vi "13_EventLogger_callback.vi"(4 "String":refnum<vi>, 5 "Event Data":cluster{"level":i32, "message":string}, 6 "Control Ref":refnum<k24>, 7 "Event Common Data":T1) -> ()   [LabVIEW 2014]
uses:
  SwabianInstruments.TimeTagger
panel:
  # "This is a callback VI that LabView will call automatically on each \ncaptured .NET Event.\n\nYou can create this VI by right clicking on \"VI Ref\" field of the \n\"Register Event Callback\" node and choosing \"Create Callback VI\""
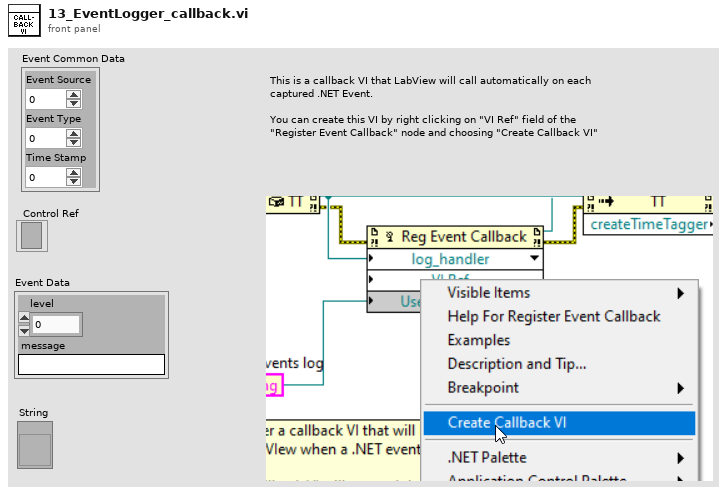
[diagram p1: front panel]
types:
  T1 = cluster{"Event Source":i32, "Event Type":u32, "Time Stamp":u32}
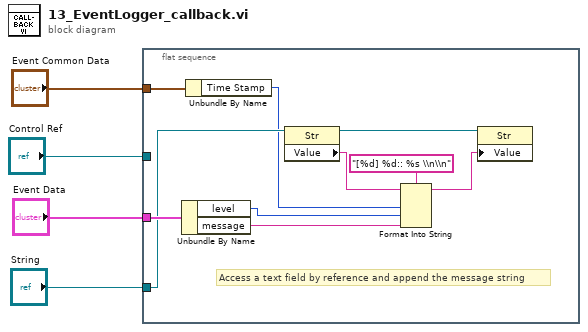
[diagram p0: block diagram]
diagram:
  n1 = flat-sequence {
    tunnel: "Event Data" -> [w14]
    tunnel: "Event Common Data" -> [w10]
    tunnel: "String" -> [w12]
    tunnel: "Control Ref" -> [_]
    frame #0 {
      # "Access a text field by reference and append the message string"
      n2 = Unbundle By Name(w14) -> ("level"=w6:i32, "message"=w5:string)
      n3 = Unbundle By Name(w10) -> ("Time Stamp"=w9:u32)
      n4 = property class="Str"(reference=w12) -> (reference out=w13:refnum<vi>, "Value"=w8:string)  [unwired: 1 in, 1 out]
      n5 = Format Into String(format string="[%d] %d:: %s \\n\\n", initial string=w8, w9, w6, w5) -> (resulting string=w7:string)  [unwired: 1 in, 1 out]
      n6 = property class="Str"(reference=w13, "Value"=w7) -> ()  [unwired: 1 in, 2 out]
    }
  }
